vi "catalog.get_ingest_progress_v2.vi"(8 "error in":errorcluster, 10 "datasetRid[]":string, 11 "Nominal Client in":refnum<class "Nominal Client.lvclass">) -> (0 "error out":errorcluster, 1 "Additional Details":T1 {"End Time" format="%<%x %.3X>T"; "Start Time" format="%<%x %.3X>T"}, 2 "Status":string, 3 "Nominal Client out":refnum<class "Nominal Client.lvclass">)   [LabVIEW 2020, in "Nominal Client.lvclass"]
uses:
  Nominal Client.lvclass
  dd643593-8eee-4817-a06c-cfd53975b380.vi
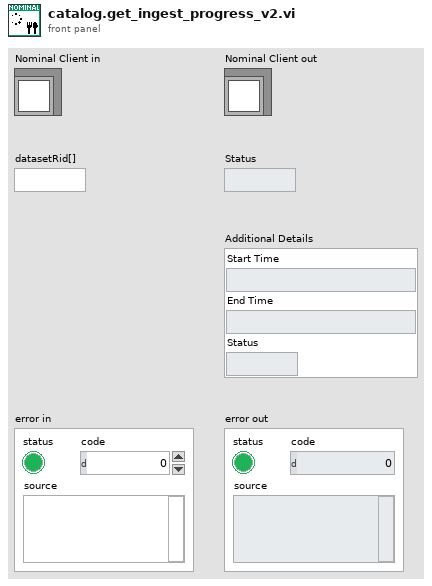
[diagram p1: front panel]
types:
  T1 = cluster{"Start Time":timestamp, "End Time":timestamp, "Status":string}
  T2 = cluster{"startTime":string, "endTime":string, "ingestStatus":cluster{"type":string, "error":cluster{"errorType":string, "message":string}}}
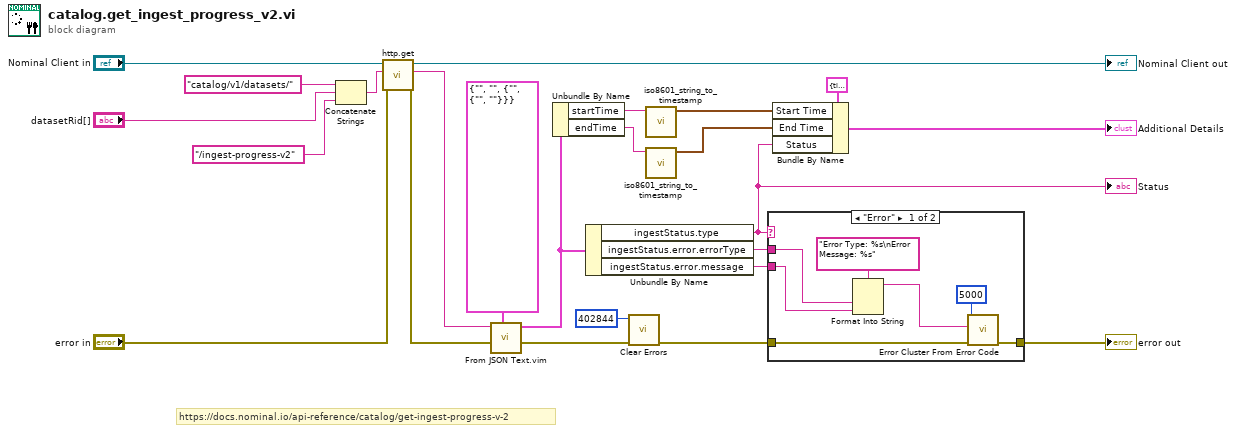
[diagram p0: block diagram]
diagram:
  # "https://docs.nominal.io/api-reference/catalog/get-ingest-progress-v-2"
  n1 = Concatenate Strings("catalog/v1/datasets/" ("Path"), "datasetRid[]", "/ingest-progress-v2" ("Path")) -> (w15:string)
  n2 = call "http.get.vi"("error in"="error in", "Path"=w15, "Nominal Client in"="Nominal Client in") -> ("error out"=w7:errorcluster, "Response"=w8:string, "Nominal Client out"=→"Nominal Client out":refnum<class "Nominal Client.lvclass">)  [unwired: 5 in, 1 out]
  n3 = call "From JSON Text.vim"("Data Type and Default Value"=T2 {"startTime"="", "endTime"="", "ingestStatus"={"type"="", "error"={"errorType"="", "message"=""}}}, "error in (no error)"=w7, "JSON"=w8) -> ("error out"=w12:errorcluster, "Data out"=w6:T2)  [unwired: 7 in]
  n4 = Unbundle By Name(w6) -> ("startTime"=w5:string, "endTime"=w4:string)
  n5 = Unbundle By Name(w6) -> ("ingestStatus.type"=w19:string, "ingestStatus.error.errorType"=w10:string, "ingestStatus.error.message"=w9:string)
  "Status" <- w19
  n6 = call <vilib>:"Clear Errors.vi"("error in (no error)"=w12, "specific error code to clear (0: all)"=402844) -> ("error out"=w11:errorcluster)  [unwired: 4 in, 1 out]
  n7 = call "iso8601_string_to_timestamp.vi"("ISO8601 Timestamp String"=w5) -> ("Time Stamp"=w2:timestamp)  [unwired: 9 in, 1 out]
  n8 = call "iso8601_string_to_timestamp.vi"("ISO8601 Timestamp String"=w4) -> ("Time Stamp"=w1:timestamp)  [unwired: 9 in, 1 out]
  n9 = case shown="\"Error\"" w19 {
    tunnel: w11 -> [w30 w32]
    tunnel: [w31 w32] -> w20
    tunnel: w10 -> [w28 _]
    tunnel: w9 -> [w27 _]
    frame "Error" {
      n10 = Format Into String(format string="Error Type: %s\nError Message: %s", w28, w27) -> (resulting string=w25:string)  [unwired: 2 in, 1 out]
      n11 = call <vilib>:"Error Cluster From Error Code.vi"("error in (no error)"=w30, "error message (\"\")"=w25, "error code (0)"=5000) -> ("error out"=w31:errorcluster)  [unwired: 6 in]
    }
    frame Default {
    }
  }
  "error out" <- w20
  n12 = Bundle By Name(cluster=T1 {"Start Time"=timestamp(0 s since 1904-01-01), "End Time"=timestamp(0 s since 1904-01-01), "Status"=""} ("Additional Details"), "Start Time"=w2, "End Time"=w1, "Status"=w19) -> (→"Additional Details":T1)
